vi "GetSglImage.vi"(8 "error in":errorcluster, 9 "Color":u32(colorbox), 10 "Height":u32, 11 "Width":u32) -> (0 "error out":errorcluster, 3 "Img":picture)   [LabVIEW 2012, in "Spinner.xctl"]
uses:
  Spinner.xctl
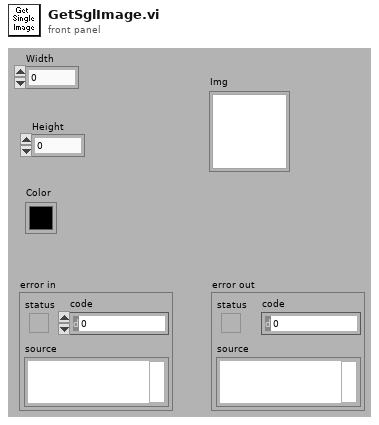
[diagram p1: front panel]
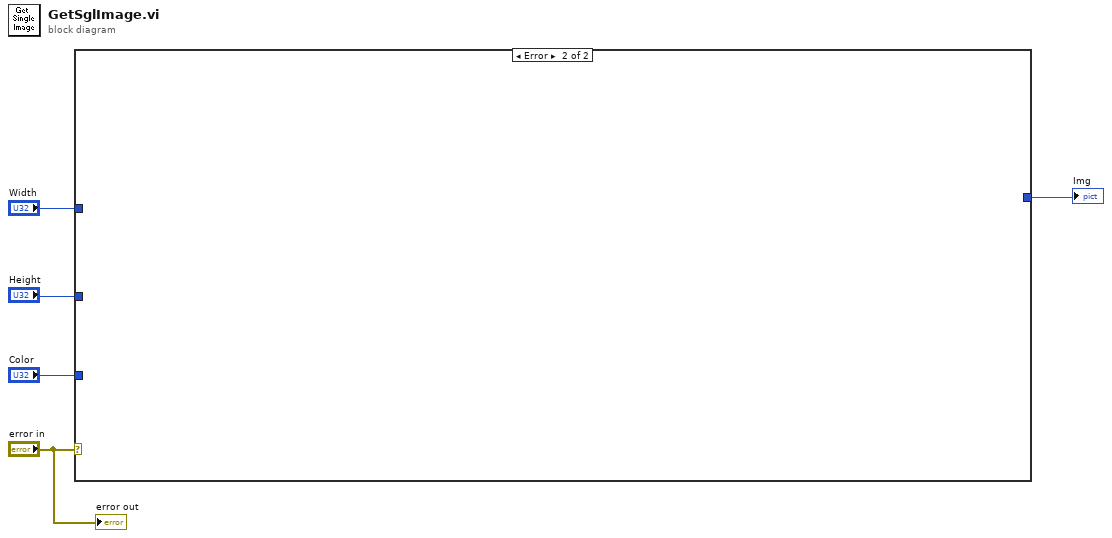
[diagram p0: block diagram]
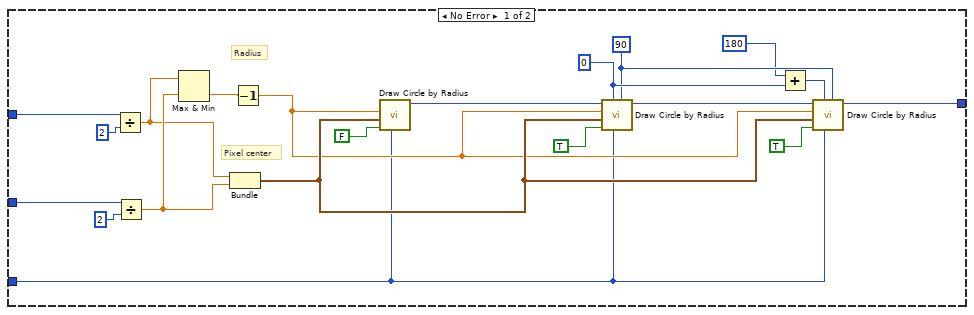
[diagram p2: hidden frame]
diagram:
  n1 = case shown="Error" "error in" {
    tunnel: "Width" -> [w9 _]
    tunnel: "Height" -> [w8 _]
    tunnel: "Color" -> [w7 _]
    tunnel: [w6 _] -> w2
    frame No Error {
      w14 = i16 90 ("arc size(360)")
      w25 = 0
      # "Radius"
      # "Pixel center"
      n2 = Divide(x=w9, y=u32 2) -> (x/y=w10:dbl)
      n3 = Divide(x=w8, y=u32 2) -> (x/y=w24:dbl)
      n4 = Max & Min(x=w10, y=w24) -> (min(x,y)=w21:dbl)  [unwired: 1 out]
      n5 = Bundle(w10, w24) -> (w20:cluster{dbl, dbl})  [unwired: 1 in]
      n6 = Decrement(x=w21) -> (x-1=w19:dbl)
      n7 = call <vilib>:"Draw Circle by Radius.vi"("color(black)"=w7, "fill?(F)"=FALSE, "pixel center"=w20, "radius"=w19) -> ("new picture"=w18:picture)  [unwired: 7 in]
      n8 = call <vilib>:"Draw Circle by Radius.vi"("arc size(360)"=w14, "color(black)"=w7, "start angle(0)"=w25, "fill?(F)"=TRUE, "pixel center"=w20, "radius"=w19, "picture"=w18) -> ("new picture"=w17:picture)  [unwired: 4 in]
      n9 = Add(x=180, y=w25) -> (x+y=w12:i32)
      n10 = call <vilib>:"Draw Circle by Radius.vi"("arc size(360)"=w14, "color(black)"=w7, "start angle(0)"=w12, "fill?(F)"=TRUE, "pixel center"=w20, "radius"=w19, "picture"=w17) -> ("new picture"=w6:picture)  [unwired: 4 in]
    }
    frame Error {
    }
  }
  "Img" <- w2
  "error out" <- "error in"
